vi "Training Top Level.vi"() -> ()   [LabVIEW 2016]
uses:
  Type Definitions/controls_setup.ctl
  Type Definitions/controls_setup_2.ctl
  Type Definitions/control_references.ctl
  <vilib>/Utility/error.llb/DialogType.ctl
panel:
  in  "Water":bool
  in  "Quit":bool=TRUE
  out "Timing Issues":bool
  in  "Config File":path=path "C:/Users/Training/Desktop/TL/lickamundo_amps.ini"
  in  "Base Directory":path=path "C:/Users/Training/Desktop/TL/batch_01_cooling_2"
  in  "Setup 3":bool
  in  "Setup 2":bool
  in  "Setup 1":bool
  in  "Setup 0":bool
  in  "S3":T1={"ChartTemp"=[{"temp in"=32.89921569824219, "temp in"=32.0}, {"temp in"=32.89724349975586, "temp in"=32.0}, {"temp in"=32.890663146972656, "temp in"=32.0}, {"temp in"=32.89329528808594, "temp in"=32.0}, {"temp in"=32.8900032043457, "temp in"=32.0}, {"temp in"=32.88868713378906, "temp in"=32.0}, {"temp in"=32.8900032043457, "temp in"=32.0}, {"temp in"=32.885398864746094, "temp in"=32.0}, {"temp in"=32.88408279418945, "temp in"=32.0}, {"temp in"=32.88079071044922, "temp in"=32.0}, {"temp in"=32.87881851196289, "temp in"=32.0}, {"temp in"=32.87092208862305, "temp in"=32.0}, {"temp in"=32.863685607910156, "temp in"=32.0}, {"temp in"=32.87355422973633, "temp in"=32.0}, {"temp in"=32.87487030029297, "temp in"=32.0}, {"temp in"=32.86763381958008, "temp in"=32.0}, {"temp in"=32.86170959472656, "temp in"=32.0}, {"temp in"=32.858421325683594, "temp in"=32.0}, {"temp in"=32.869606018066406, "temp in"=32.0}, {"temp in"=32.87026596069336, "temp in"=32.0}, {"temp in"=32.865657806396484, "temp in"=32.0}, {"temp in"=32.865657806396484, "temp in"=32.0}, {"temp in"=32.861053466796875, "temp in"=32.0}, {"temp in"=32.863685607910156, "temp in"=32.0}, {"temp in"=32.86170959472656, "temp in"=32.0}, {"temp in"=32.865657806396484, "temp in"=32.0}, {"temp in"=32.862369537353516, "temp in"=32.0}, {"temp in"=32.85578918457031, "temp in"=32.0}, {"temp in"=32.85907745361328, "temp in"=32.0}, {"temp in"=32.8564453125, "temp in"=32.0}, {"temp in"=32.845916748046875, "temp in"=32.0}, {"temp in"=32.85710525512695, "temp in"=32.0}, {"temp in"=32.85249710083008, "temp in"=32.0}, {"temp in"=32.85315704345703, "temp in"=32.0}, {"temp in"=32.85052490234375, "temp in"=32.0}, {"temp in"=32.85447311401367, "temp in"=32.0}, {"temp in"=32.85512924194336, "temp in"=32.0}, {"temp in"=32.86170959472656, "temp in"=32.0}, {"temp in"=32.87487030029297, "temp in"=32.0}, {"temp in"=32.8900032043457, "temp in"=32.0}, {"temp in"=32.906455993652344, "temp in"=32.0}, {"temp in"=32.91303634643555, "temp in"=32.0}, {"temp in"=32.92816925048828, "temp in"=32.0}, {"temp in"=32.93935775756836, "temp in"=32.0}, {"temp in"=32.94659423828125, "temp in"=32.0}, {"temp in"=32.87553024291992, "temp in"=32.0}, {"temp in"=32.891319274902344, "temp in"=32.0}, {"temp in"=32.864341735839844, "temp in"=32.0}, {"temp in"=32.843284606933594, "temp in"=32.0}, {"temp in"=32.844600677490234, "temp in"=32.0}], "ChartLick"=[0.22792984545230865, 0.22776533663272858, 0.22727182507514954, 0.22710731625556946, 0.22644929587841034, 0.2259557843208313, 0.22562678158283234, 0.22529776394367218, 0.22496876120567322, 0.22463975846767426, 0.22463975846767426, 0.2243107408285141, 0.22381722927093506, 0.2234882265329361, 0.22283020615577698, 0.22233669459819794, 0.2218431830406189, 0.2210206538438797, 0.22069165110588074, 0.21986912190914154, 0.21970462799072266, 0.2193756103515625, 0.21888209879398346, 0.21871758997440338, 0.2185530960559845, 0.21805958449840546, 0.2177305668592453, 0.2177305668592453, 0.21756607294082642, 0.21756607294082642, 0.21723705530166626, 0.21674354374408722, 0.21657903492450714, 0.2160855233669281, 0.21592102944850922, 0.21559201180934906, 0.21542751789093018, 0.21542751789093018, 0.21542751789093018, 0.21559201180934906, 0.21625003218650818, 0.21674354374408722, 0.21805958449840546, 0.2193756103515625, 0.22085615992546082, 0.22250120341777802, 0.22365272045135498, 0.2243107408285141, 0.22447524964809418, 0.22447524964809418], "Catch Trials"={"Catch Trials"=0, "Correct Rejections"=0, "False Alarms"=0, "Performance"=100}, "DispStim"={"n"=0, "Hits"=0, "Misses"=0, "Performance"=0}, "Bools"={"Stimulus"=FALSE, "Catch"=FALSE, "Square"=FALSE, "Lick"=FALSE, "Water"=FALSE}, "Time to next stimulus"=0.0, "Recording"=FALSE} {"Time to next stimulus" scale=0.0..1000.0; "DispStim"."Performance" format="%d%%"; "Catch Trials"."Performance" format="%d%%"}
  in  "S2":T1={"ChartTemp"=[{"temp in"=31.964832305908203, "temp in"=32.0}, {"temp in"=31.966148376464844, "temp in"=32.0}, {"temp in"=31.966148376464844, "temp in"=32.0}, {"temp in"=31.970096588134766, "temp in"=32.0}, {"temp in"=31.973386764526367, "temp in"=32.0}, {"temp in"=31.968780517578125, "temp in"=32.0}, {"temp in"=31.968122482299805, "temp in"=32.0}, {"temp in"=31.964174270629883, "temp in"=32.0}, {"temp in"=31.971412658691406, "temp in"=32.0}, {"temp in"=31.969438552856445, "temp in"=32.0}, {"temp in"=31.970096588134766, "temp in"=32.0}, {"temp in"=31.969438552856445, "temp in"=32.0}, {"temp in"=31.970096588134766, "temp in"=32.0}, {"temp in"=31.970096588134766, "temp in"=32.0}, {"temp in"=31.970754623413086, "temp in"=32.0}, {"temp in"=31.972728729248047, "temp in"=32.0}, {"temp in"=31.974044799804688, "temp in"=32.0}, {"temp in"=31.974044799804688, "temp in"=32.0}, {"temp in"=31.972070693969727, "temp in"=32.0}, {"temp in"=31.972728729248047, "temp in"=32.0}, {"temp in"=31.971412658691406, "temp in"=32.0}, {"temp in"=31.970754623413086, "temp in"=32.0}, {"temp in"=31.970754623413086, "temp in"=32.0}, {"temp in"=31.974044799804688, "temp in"=32.0}, {"temp in"=31.972728729248047, "temp in"=32.0}, {"temp in"=31.972728729248047, "temp in"=32.0}, {"temp in"=31.968122482299805, "temp in"=32.0}, {"temp in"=31.968780517578125, "temp in"=32.0}, {"temp in"=31.967464447021484, "temp in"=32.0}, {"temp in"=31.973386764526367, "temp in"=32.0}, {"temp in"=31.970754623413086, "temp in"=32.0}, {"temp in"=31.970096588134766, "temp in"=32.0}, {"temp in"=31.968780517578125, "temp in"=32.0}, {"temp in"=31.968122482299805, "temp in"=32.0}, {"temp in"=31.970754623413086, "temp in"=32.0}, {"temp in"=31.967464447021484, "temp in"=32.0}, {"temp in"=31.969438552856445, "temp in"=32.0}, {"temp in"=31.970096588134766, "temp in"=32.0}, {"temp in"=31.970096588134766, "temp in"=32.0}, {"temp in"=31.968122482299805, "temp in"=32.0}, {"temp in"=31.965490341186523, "temp in"=32.0}, {"temp in"=31.967464447021484, "temp in"=32.0}, {"temp in"=31.966806411743164, "temp in"=32.0}, {"temp in"=31.968780517578125, "temp in"=32.0}, {"temp in"=31.970096588134766, "temp in"=32.0}, {"temp in"=31.965490341186523, "temp in"=32.0}, {"temp in"=31.967464447021484, "temp in"=32.0}, {"temp in"=31.968122482299805, "temp in"=32.0}, {"temp in"=31.968780517578125, "temp in"=32.0}, {"temp in"=31.969438552856445, "temp in"=32.0}], "ChartLick"=[-0.029354939237236977, -0.029354939237236977, -0.029519444331526756, -0.029848452657461166, -0.029848452657461166, -0.030341966077685356, -0.030177460983395576, -0.030506469309329987, -0.030506469309329987, -0.030341966077685356, -0.030670974403619766, -0.030670974403619766, -0.030341966077685356, -0.030506469309329987, -0.030177460983395576, -0.029848452657461166, -0.029848452657461166, -0.029519444331526756, -0.029354939237236977, -0.029354939237236977, -0.029190434142947197, -0.029190434142947197, -0.029354939237236977, -0.029190434142947197, -0.029190434142947197, -0.029519444331526756, -0.029190434142947197, -0.029354939237236977, -0.029354939237236977, -0.029190434142947197, -0.028861425817012787, -0.028861425817012787, -0.029025930911302567, -0.029190434142947197, -0.029025930911302567, -0.029354939237236977, -0.029354939237236977, -0.029519444331526756, -0.029683947563171387, -0.029519444331526756, -0.029354939237236977, -0.029354939237236977, -0.029190434142947197, -0.029190434142947197, -0.029190434142947197, -0.028861425817012787, -0.029354939237236977, -0.029354939237236977, -0.029519444331526756, -0.029683947563171387], "Catch Trials"={"Catch Trials"=0, "Correct Rejections"=0, "False Alarms"=0, "Performance"=100}, "DispStim"={"n"=0, "Hits"=0, "Misses"=0, "Performance"=0}, "Bools"={"Stimulus"=FALSE, "Catch"=FALSE, "Square"=FALSE, "Lick"=FALSE, "Water"=FALSE}, "Time to next stimulus"=0.0, "Recording"=FALSE} {"Time to next stimulus" scale=0.0..1000.0; "DispStim"."Performance" format="%d%%"; "Catch Trials"."Performance" format="%d%%"}
  in  "S1":T1={"ChartTemp"=[{"temp in"=31.926668167114258, "temp in"=32.0}, {"temp in"=31.93785285949707, "temp in"=32.0}, {"temp in"=31.93456268310547, "temp in"=32.0}, {"temp in"=31.926668167114258, "temp in"=32.0}, {"temp in"=31.92930030822754, "temp in"=32.0}, {"temp in"=31.926010131835938, "temp in"=32.0}, {"temp in"=31.93587875366211, "temp in"=32.0}, {"temp in"=31.927326202392578, "temp in"=32.0}, {"temp in"=31.93719482421875, "temp in"=32.0}, {"temp in"=31.92995834350586, "temp in"=32.0}, {"temp in"=31.947065353393555, "temp in"=32.0}, {"temp in"=31.92995834350586, "temp in"=32.0}, {"temp in"=31.92864227294922, "temp in"=32.0}, {"temp in"=31.93653678894043, "temp in"=32.0}, {"temp in"=31.93785285949707, "temp in"=32.0}, {"temp in"=31.93390655517578, "temp in"=32.0}, {"temp in"=31.93456268310547, "temp in"=32.0}, {"temp in"=31.93851089477539, "temp in"=32.0}, {"temp in"=31.93916893005371, "temp in"=32.0}, {"temp in"=31.93522071838379, "temp in"=32.0}, {"temp in"=31.93193244934082, "temp in"=32.0}, {"temp in"=31.93456268310547, "temp in"=32.0}, {"temp in"=31.93785285949707, "temp in"=32.0}, {"temp in"=31.93916893005371, "temp in"=32.0}, {"temp in"=31.94048500061035, "temp in"=32.0}, {"temp in"=31.944433212280273, "temp in"=32.0}, {"temp in"=31.945749282836914, "temp in"=32.0}, {"temp in"=31.93390655517578, "temp in"=32.0}, {"temp in"=31.93324851989746, "temp in"=32.0}, {"temp in"=31.941143035888672, "temp in"=32.0}, {"temp in"=31.941143035888672, "temp in"=32.0}, {"temp in"=31.945091247558594, "temp in"=32.0}, {"temp in"=31.93851089477539, "temp in"=32.0}, {"temp in"=31.93061637878418, "temp in"=32.0}, {"temp in"=31.93587875366211, "temp in"=32.0}, {"temp in"=31.925352096557617, "temp in"=32.0}, {"temp in"=31.941143035888672, "temp in"=32.0}, {"temp in"=31.947723388671875, "temp in"=32.0}, {"temp in"=31.946407318115234, "temp in"=32.0}, {"temp in"=31.93916893005371, "temp in"=32.0}, {"temp in"=31.942459106445312, "temp in"=32.0}, {"temp in"=31.93916893005371, "temp in"=32.0}, {"temp in"=31.93916893005371, "temp in"=32.0}, {"temp in"=31.93785285949707, "temp in"=32.0}, {"temp in"=31.93259048461914, "temp in"=32.0}, {"temp in"=31.947065353393555, "temp in"=32.0}, {"temp in"=31.94048500061035, "temp in"=32.0}, {"temp in"=31.94048500061035, "temp in"=32.0}, {"temp in"=31.93522071838379, "temp in"=32.0}, {"temp in"=31.93851089477539, "temp in"=32.0}], "ChartLick"=[-0.015372068621218204, 0.008645567111670971, 0.010455114766955376, 0.01226466242223978, 0.01308718416839838, 0.32400035858154297, 0.4118456542491913, 0.3945727050304413, 0.2456963062286377, 0.11310582607984543, 0.023286454379558563, -0.004679285921156406, -0.002376224845647812, -0.0031987465918064117, -0.0033632509876042604, -0.30802538990974426, -0.4100181758403778, -0.41363725066185, -0.26953136920928955, -0.12542548775672913, -0.01553657278418541, 0.008810071274638176, 0.01111313235014677, 0.012100158259272575, 0.012100158259272575, 0.32498738169670105, 0.4116811454296112, 0.3906245827674866, 0.24306423962116241, 0.11491537094116211, 0.021312402561306953, -0.004514781292527914, -0.0027052334044128656, -0.002540729008615017, -0.0033632509876042604, -0.3095059394836426, -0.4108406901359558, -0.4123212397098541, -0.2677218019962311, -0.12493197619915009, -0.015207564458251, 0.008645567111670971, 0.011277636513113976, 0.012100158259272575, 0.012429166585206985, 0.3287709653377533, 0.40970709919929504, 0.3934211730957031, 0.24372224509716034, 0.11195429414510727], "Catch Trials"={"Catch Trials"=135, "Correct Rejections"=0, "False Alarms"=135, "Performance"=0}, "DispStim"={"n"=136, "Hits"=136, "Misses"=0, "Performance"=100}, "Bools"={"Stimulus"=FALSE, "Catch"=FALSE, "Square"=FALSE, "Lick"=FALSE, "Water"=FALSE}, "Time to next stimulus"=20000.0, "Recording"=FALSE} caption="Setup 1" {"Time to next stimulus" scale=0.0..20000.0; "DispStim"."Performance" format="%d%%"; "Catch Trials"."Performance" format="%d%%"}
  in  "S0":T1={"ChartTemp"=[{"temp in"=31.942459106445312, "temp in"=32.0}, {"temp in"=31.951013565063477, "temp in"=32.0}, {"temp in"=31.949697494506836, "temp in"=32.0}, {"temp in"=31.949039459228516, "temp in"=32.0}, {"temp in"=31.951013565063477, "temp in"=32.0}, {"temp in"=31.950355529785156, "temp in"=32.0}, {"temp in"=31.95890998840332, "temp in"=32.0}, {"temp in"=31.944433212280273, "temp in"=32.0}, {"temp in"=31.952987670898438, "temp in"=32.0}, {"temp in"=31.945749282836914, "temp in"=32.0}, {"temp in"=31.92995834350586, "temp in"=32.0}, {"temp in"=31.954303741455078, "temp in"=32.0}, {"temp in"=31.943117141723633, "temp in"=32.0}, {"temp in"=31.95956802368164, "temp in"=32.0}, {"temp in"=31.962858200073242, "temp in"=32.0}, {"temp in"=31.9615421295166, "temp in"=32.0}, {"temp in"=31.9615421295166, "temp in"=32.0}, {"temp in"=31.9615421295166, "temp in"=32.0}, {"temp in"=31.962200164794922, "temp in"=32.0}, {"temp in"=31.966148376464844, "temp in"=32.0}, {"temp in"=31.96088409423828, "temp in"=32.0}, {"temp in"=31.95759391784668, "temp in"=32.0}, {"temp in"=31.954303741455078, "temp in"=32.0}, {"temp in"=31.962858200073242, "temp in"=32.0}, {"temp in"=31.962200164794922, "temp in"=32.0}, {"temp in"=31.952329635620117, "temp in"=32.0}, {"temp in"=31.94048500061035, "temp in"=32.0}, {"temp in"=31.95759391784668, "temp in"=32.0}, {"temp in"=31.952987670898438, "temp in"=32.0}, {"temp in"=31.966806411743164, "temp in"=32.0}, {"temp in"=31.958251953125, "temp in"=32.0}, {"temp in"=31.95890998840332, "temp in"=32.0}, {"temp in"=31.962858200073242, "temp in"=32.0}, {"temp in"=31.95956802368164, "temp in"=32.0}, {"temp in"=31.9549617767334, "temp in"=32.0}, {"temp in"=31.9549617767334, "temp in"=32.0}, {"temp in"=31.964174270629883, "temp in"=32.0}, {"temp in"=31.95759391784668, "temp in"=32.0}, {"temp in"=31.962858200073242, "temp in"=32.0}, {"temp in"=31.96088409423828, "temp in"=32.0}, {"temp in"=31.95759391784668, "temp in"=32.0}, {"temp in"=31.95627784729004, "temp in"=32.0}, {"temp in"=31.966806411743164, "temp in"=32.0}, {"temp in"=31.95693588256836, "temp in"=32.0}, {"temp in"=31.95890998840332, "temp in"=32.0}, {"temp in"=31.966148376464844, "temp in"=32.0}, {"temp in"=31.96088409423828, "temp in"=32.0}, {"temp in"=31.95627784729004, "temp in"=32.0}, {"temp in"=31.972070693969727, "temp in"=32.0}, {"temp in"=31.958251953125, "temp in"=32.0}], "ChartLick"=[-0.019978191703557968, 0.008974575437605381, 0.010948628187179565, 0.011771149933338165, 0.013251688331365585, 0.32021674513816833, 0.41299718618392944, 0.39555972814559937, 0.2440512627363205, 0.11524438112974167, 0.021147897467017174, -0.0050082942470908165, -0.0027052334044128656, -0.003034242196008563, -0.0033632509876042604, -0.3034192621707916, -0.4126502275466919, -0.4157758355140686, -0.2718344032764435, -0.1272350400686264, -0.01586558111011982, 0.008481062948703766, 0.010948628187179565, 0.011771149933338165, 0.01275817584246397, 0.3190652132034302, 0.4125036597251892, 0.39309215545654297, 0.24207721650600433, 0.11606690287590027, 0.023286454379558563, -0.004514781292527914, -0.002376224845647812, -0.0028697378002107143, -0.003692259546369314, -0.3075318932533264, -0.4108406901359558, -0.41314375400543213, -0.266734778881073, -0.12855108082294464, -0.01553657278418541, 0.008974575437605381, 0.01111313235014677, 0.011771149933338165, 0.012429166585206985, 0.32416486740112305, 0.4106941223144531, 0.3934211730957031, 0.2448737770318985, 0.11343482881784439], "Catch Trials"={"Catch Trials"=115, "Correct Rejections"=0, "False Alarms"=115, "Performance"=0}, "DispStim"={"n"=116, "Hits"=116, "Misses"=0, "Performance"=100}, "Bools"={"Stimulus"=FALSE, "Catch"=FALSE, "Square"=FALSE, "Lick"=FALSE, "Water"=FALSE}, "Time to next stimulus"=20000.0, "Recording"=FALSE} {"Time to next stimulus" scale=0.0..20000.0; "DispStim"."Performance" format="%d%%"; "Catch Trials"."Performance" format="%d%%"}
  in  "Setup 3 Controls":T2={"Animal"=4, "Session"=1, "Free Reward"=FALSE, "Start"=FALSE, "Pause"=FALSE, "Stop"=FALSE} {"Session" min=1 step=1 format="%03.0f"; "Animal" min=1 step=1 format="%03.0f"}
  in  "Setup 2 Controls":T2={"Animal"=3, "Session"=2, "Free Reward"=FALSE, "Start"=FALSE, "Pause"=FALSE, "Stop"=FALSE} {"Session" min=1 step=1 format="%03.0f"; "Animal" min=1 step=1 format="%03.0f"}
  in  "Setup 1 Controls":T2={"Animal"=2, "Session"=6, "Free Reward"=FALSE, "Start"=FALSE, "Pause"=FALSE, "Stop"=FALSE} {"Session" min=1 step=1 format="%03.0f"; "Animal" min=1 step=1 format="%03.0f"}
  in  "Setup 0 Controls":T2={"Animal"=3, "Session"=3, "Free Reward"=FALSE, "Start"=FALSE, "Pause"=FALSE, "Stop"=FALSE} {"Session" min=1 step=1 format="%03.0f"; "Animal" min=1 step=1 format="%03.0f"}
  # "Animal Training"
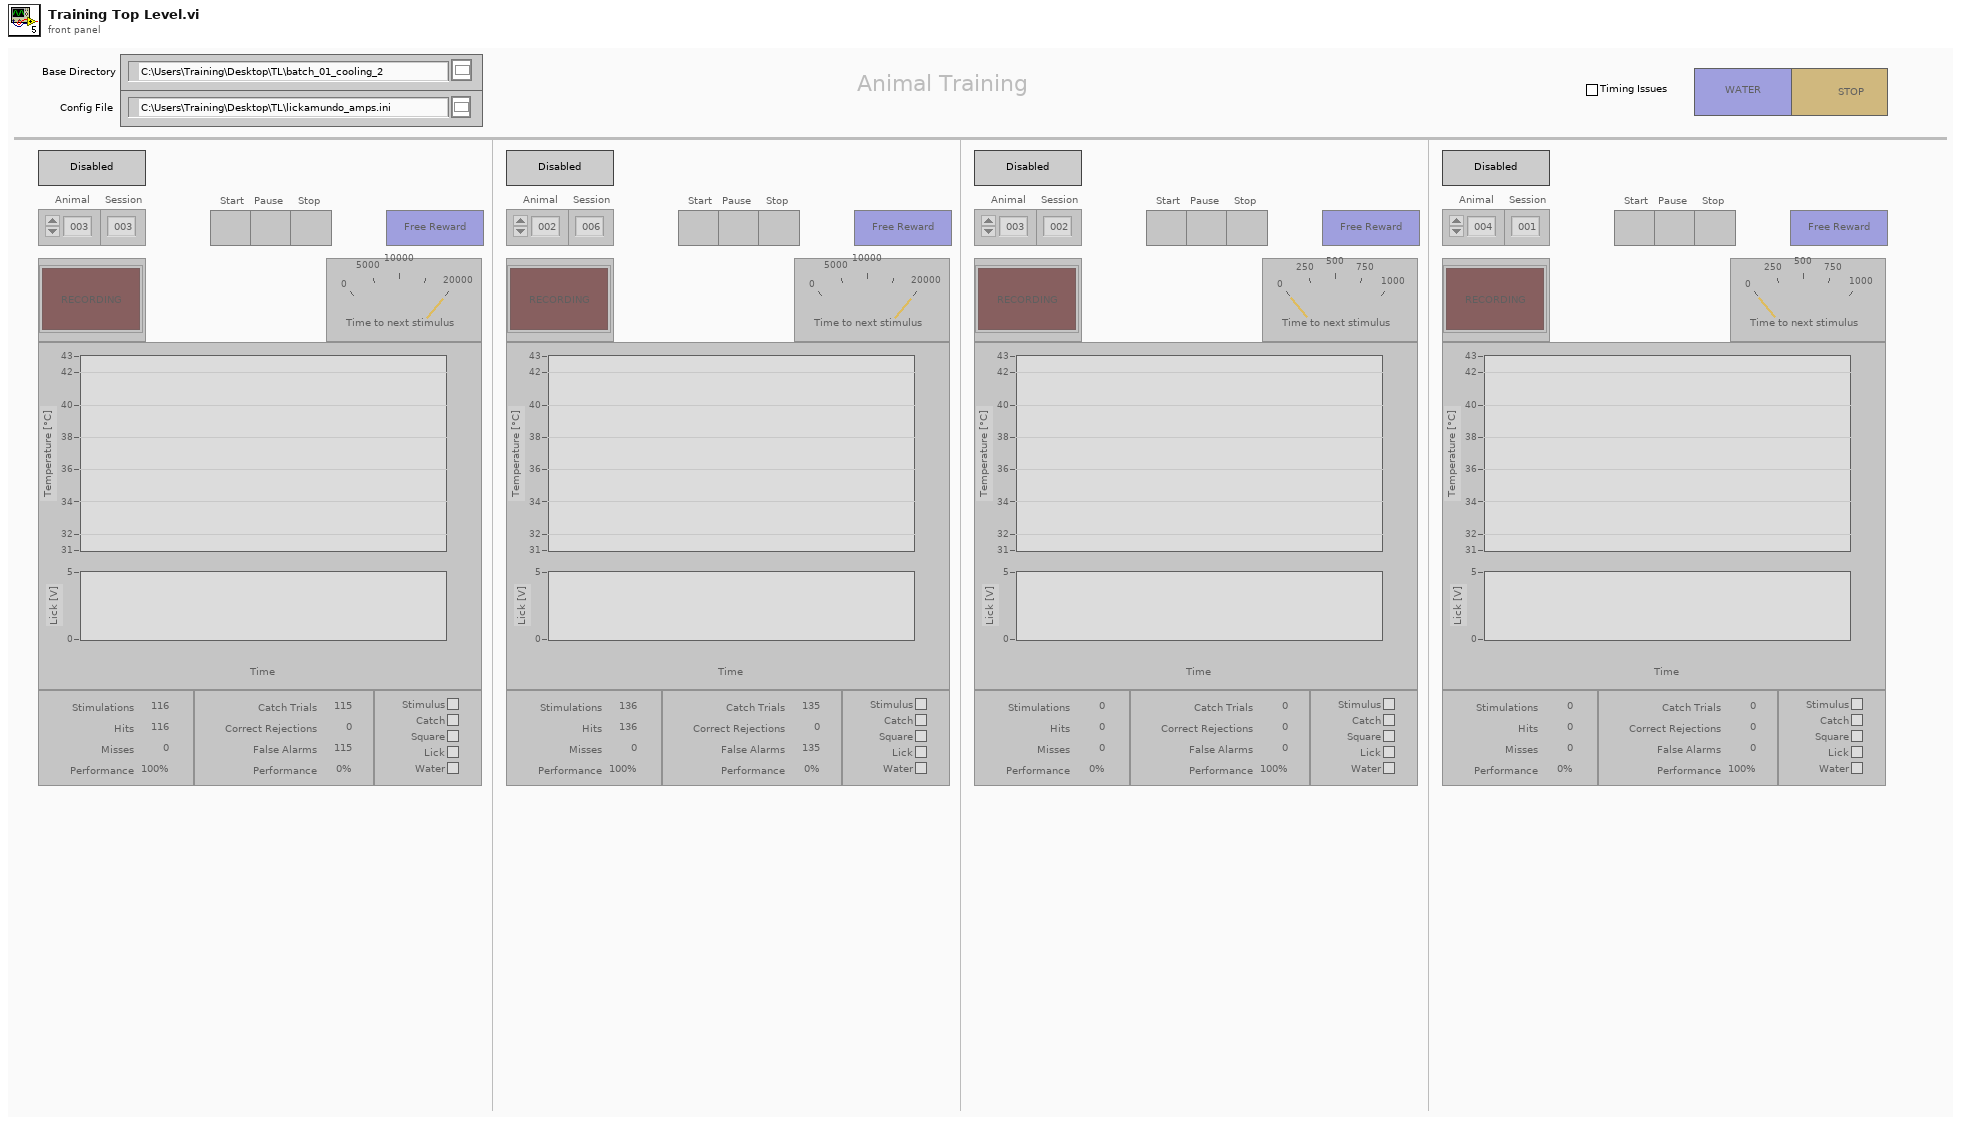
[diagram p1: front panel]
types:
  T1 = typedef "controls_setup.ctl" = cluster{"ChartTemp":cluster{"temp in":dbl, "temp in":dbl}[], "ChartLick":dbl[], "Catch Trials":cluster{"Catch Trials":u16, "Correct Rejections":u16, "False Alarms":u16, "Performance":u16}, "DispStim":cluster{"n":u16, "Hits":u16, "Misses":u16, "Performance":u16}, "Bools":cluster{"Stimulus":bool, "Catch":bool, "Square":bool, "Lick":bool, "Water":bool}, "Time to next stimulus":dbl, "Recording":bool}
  T2 = typedef "controls_setup_2.ctl" = cluster{"Animal":u16, "Session":u16, "Free Reward":bool, "Start":bool, "Pause":bool, "Stop":bool}
  T3 = typedef "DialogType.ctl" = u16
  T4 = typedef "control_references.ctl" = cluster{"Base Directory":refnum<vi>, "Config File":refnum<vi>, "Timing Issues":refnum<vi>, "Quit":refnum<vi>, "Animal ID":refnum<vi>[], "Session ID":refnum<vi>[], "Active":refnum<vi>[], "Temperature Charts":refnum<vi>[], "Lick Charts":refnum<vi>[], "Bool Displays":refnum<vi>[], "Stimulus Timing":refnum<vi>[], "Stimulus Stats":refnum<vi>[], "Catch Stats":refnum<vi>[], "Recording Status":refnum<vi>[]}
  T5 = typedef "reference_cluster.ctl" = cluster{"Vars":cluster{"General":refnum<notifier>, "Runtime":refnum<notifier>}, "Data":cluster{"Display":refnum<queue>, "Write":refnum<queue>}, "LoopCtrl":cluster{"Display":refnum<notifier>, "DAQ":refnum<notifier>, "Write":refnum<notifier>[]}, "Controls":T4, "Error Event":refnum<user-event>}
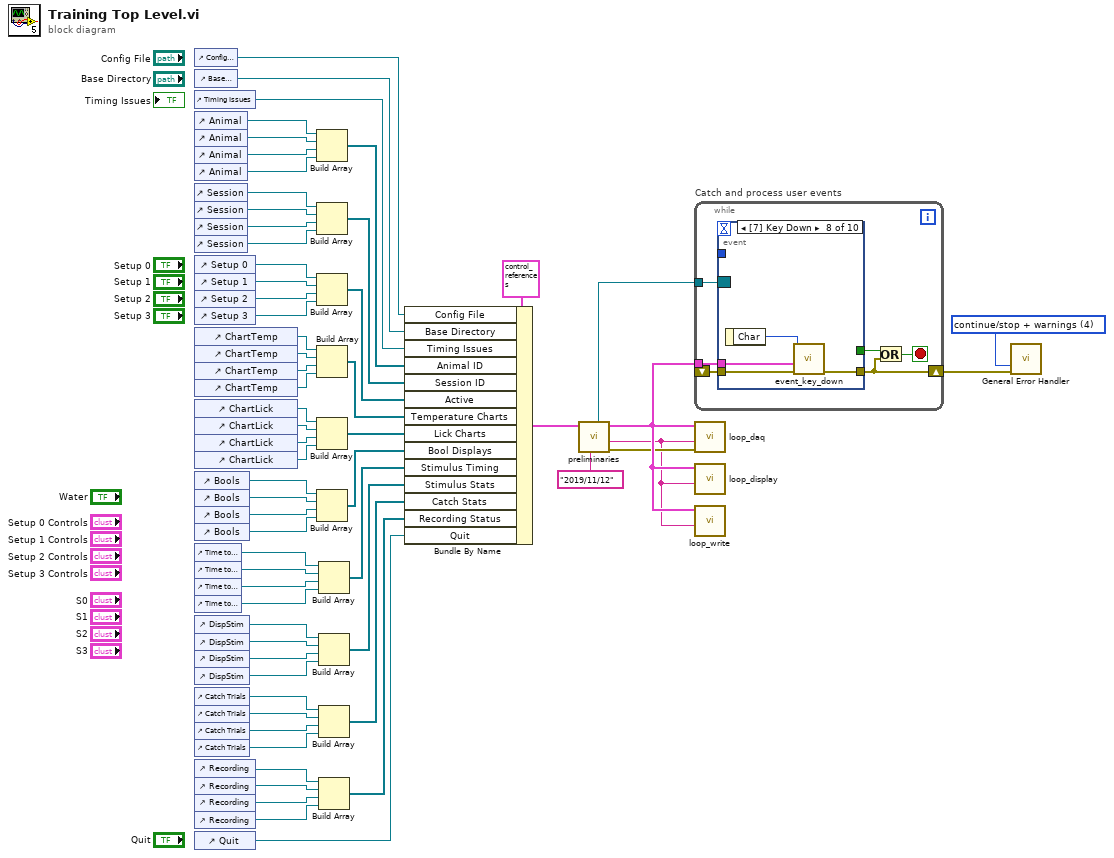
[diagram p0: block diagram]
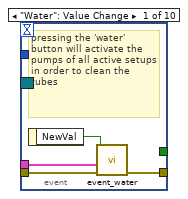
[diagram p2: hidden frame]
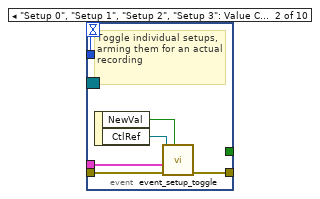
[diagram p3: hidden frame]
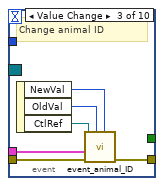
[diagram p4: hidden frame]
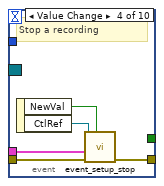
[diagram p5: hidden frame]
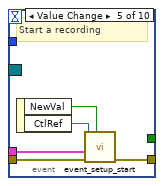
[diagram p6: hidden frame]
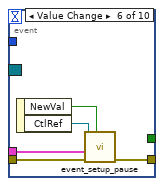
[diagram p7: hidden frame]
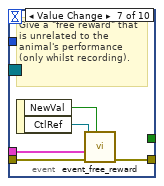
[diagram p8: hidden frame]
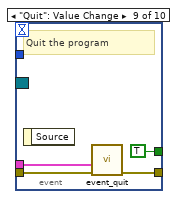
[diagram p9: hidden frame]
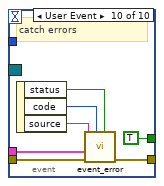
[diagram p10: hidden frame]
diagram:
  w10 = T3 4 items=["no dialog", "OK message", "continue or stop message", "OK message + warnings", "continue/stop + warnings"] ("type of dialog (OK msg:1)")
  n1 = control-ref of="Config File"() -> (w13:refnum<vi>)
  n2 = control-ref of="Base Directory"() -> (w38:refnum<vi>)
  n3 = control-ref of="Timing Issues"() -> (w39:refnum<vi>)
  n4 = control-ref of="Animal"() -> (w37:refnum<vi>)
  n5 = control-ref of="Animal"() -> (w36:refnum<vi>)
  n6 = control-ref of="Animal"() -> (w35:refnum<vi>)
  n7 = control-ref of="Animal"() -> (w34:refnum<vi>)
  n8 = control-ref of="Session"() -> (w33:refnum<vi>)
  n9 = control-ref of="Session"() -> (w32:refnum<vi>)
  n10 = control-ref of="Session"() -> (w31:refnum<vi>)
  n11 = control-ref of="Session"() -> (w30:refnum<vi>)
  n12 = control-ref of="Setup 0"() -> (w29:refnum<vi>)
  n13 = control-ref of="Setup 1"() -> (w28:refnum<vi>)
  n14 = control-ref of="Setup 2"() -> (w27:refnum<vi>)
  n15 = control-ref of="Setup 3"() -> (w26:refnum<vi>)
  n16 = control-ref of="ChartTemp"() -> (w62:refnum<vi>)
  n17 = control-ref of="ChartTemp"() -> (w61:refnum<vi>)
  n18 = control-ref of="ChartTemp"() -> (w60:refnum<vi>)
  n19 = control-ref of="ChartTemp"() -> (w59:refnum<vi>)
  n20 = control-ref of="ChartLick"() -> (w58:refnum<vi>)
  n21 = control-ref of="ChartLick"() -> (w55:refnum<vi>)
  n22 = control-ref of="ChartLick"() -> (w56:refnum<vi>)
  n23 = control-ref of="ChartLick"() -> (w57:refnum<vi>)
  n24 = control-ref of="Bools"() -> (w54:refnum<vi>)
  n25 = control-ref of="Bools"() -> (w51:refnum<vi>)
  n26 = control-ref of="Bools"() -> (w52:refnum<vi>)
  n27 = control-ref of="Bools"() -> (w53:refnum<vi>)
  n28 = control-ref of="Time to next stimulus"() -> (w50:refnum<vi>)
  n29 = control-ref of="Time to next stimulus"() -> (w47:refnum<vi>)
  n30 = control-ref of="Time to next stimulus"() -> (w48:refnum<vi>)
  n31 = control-ref of="Time to next stimulus"() -> (w49:refnum<vi>)
  n32 = control-ref of="DispStim"() -> (w25:refnum<vi>)
  n33 = control-ref of="DispStim"() -> (w23:refnum<vi>)
  n34 = control-ref of="DispStim"() -> (w22:refnum<vi>)
  n35 = control-ref of="DispStim"() -> (w24:refnum<vi>)
  n36 = control-ref of="Catch Trials"() -> (w18:refnum<vi>)
  n37 = control-ref of="Catch Trials"() -> (w20:refnum<vi>)
  n38 = control-ref of="Catch Trials"() -> (w21:refnum<vi>)
  n39 = control-ref of="Catch Trials"() -> (w19:refnum<vi>)
  n40 = control-ref of="Recording"() -> (w9:refnum<vi>)
  n41 = control-ref of="Recording"() -> (w8:refnum<vi>)
  n42 = control-ref of="Recording"() -> (w7:refnum<vi>)
  n43 = control-ref of="Recording"() -> (w6:refnum<vi>)
  n44 = control-ref of="Quit"() -> (w12:refnum<vi>)
  n45 = Build Array(w37, w36, w35, w34) -> (w40:refnum<vi>[])
  n46 = Build Array(w33, w32, w31, w30) -> (w41:refnum<vi>[])
  n47 = Build Array(w29, w28, w27, w26) -> (w44:refnum<vi>[])
  n48 = Build Array(w62, w61, w60, w59) -> (w46:refnum<vi>[])
  n49 = Build Array(w58, w55, w56, w57) -> (w45:refnum<vi>[])
  n50 = Build Array(w54, w51, w52, w53) -> (w14:refnum<vi>[])
  n51 = Build Array(w50, w47, w48, w49) -> (w43:refnum<vi>[])
  n52 = Build Array(w25, w23, w22, w24) -> (w17:refnum<vi>[])
  n53 = Build Array(w18, w20, w21, w19) -> (w16:refnum<vi>[])
  n54 = Build Array(w9, w8, w7, w6) -> (w15:refnum<vi>[])
  n55 = Bundle By Name(cluster=T4 {"Base Directory"=refnum, "Config File"=refnum, "Timing Issues"=refnum, "Quit"=refnum, "Animal ID"=[], "Session ID"=[], "Active"=[], "Temperature Charts"=[], "Lick Charts"=[], "Bool Displays"=[], "Stimulus Timing"=[], "Stimulus Stats"=[], "Catch Stats"=[], "Recording Status"=[]} ("Cluster"), "Config File"=w13, "Base Directory"=w38, "Timing Issues"=w39, "Animal ID"=w40, "Session ID"=w41, "Active"=w44, "Temperature Charts"=w46, "Lick Charts"=w45, "Bool Displays"=w14, "Stimulus Timing"=w43, "Stimulus Stats"=w17, "Catch Stats"=w16, "Recording Status"=w15, "Quit"=w12) -> (w1:T4)
  n56 = call "preliminaries.vi"("Version"="2019/11/12" ("Last modified"), "control cluster"=w1) -> ("error out"=w5:errorcluster, "timing source out"=w4:string, "reference cluster out"=w63:T5, "error event refnum"=w2:refnum<event-registration>)  [unwired: 4 in]
  n57 = while "Catch and process user events" {
    shift-right: [w65] -> w11
    shift-left: _ -> [w69]
    tunnel: w63 -> [w68]
    tunnel: w2 -> [w64]
    stop <- w67 stop-if-true
    n58 = event shown="[7] Key Down" {
      selector: w64 -> [_ _ _ _ _ _ _ _ _ _]
      dyn-events: _ -> [_ _ _ _ _ _ _ _ _ _]
      timeout: _ -> [_ w74 _ _ _ _ _ _ _ _]
      tunnel: [_ _ _ _ _ _ _ _ TRUE TRUE] -> w66
      tunnel: w69 -> [w72 w76 w85 w88 w93 w99 w105 w109 w112 w119]
      tunnel: [w73 w79 w84 w90 w95 w98 w104 w108 w111 w120] -> w65
      tunnel: w68 -> [w71 w78 w80 w89 w94 w100 w103 w106 w110 w118]
      tunnel: [_ w74 _ _ _ _ _ _ _ _] -> _
      event "Water": Value Change {
        # "pressing the 'water' button will activate the pumps of all active setups in order to clean the tubes"
        n59 = event-data() -> ("NewVal"=w70:bool)  [unwired: 1 in]
        n60 = call "event_water.vi"("error in"=w72, "reference cluster in"=w71, "water on?"=w70) -> ("error out"=w73:errorcluster)  [unwired: 8 in]
      }
      event "Setup 0", "Setup 1", "Setup 2", "Setup 3": Value Change {
        # "Toggle individual setups, arming them for an actual recording"
        n61 = event-data() -> ("NewVal"=w75:bool, "CtlRef"=w77:refnum<vi>)  [unwired: 1 in]
        n62 = call "event_setup_toggle.vi"("NewVal"=w75, "error in"=w76, "reference cluster in"=w78, "Boolean in"=w77) -> ("error out"=w79:errorcluster)  [unwired: 7 in]
      }
      event Value Change {
        # "Change animal ID"
        n63 = event-data() -> ("NewVal"=w81:u16, "OldVal"=w82:u16, "CtlRef"=w83:refnum<vi>)  [unwired: 1 in]
        n64 = call "event_animal_ID.vi"("NewVal"=w81, "OldVal"=w82, "error in"=w85, "reference cluster in"=w80, "Digital in"=w83) -> ("error out"=w84:errorcluster)  [unwired: 6 in]
      }
      event Value Change {
        # "Stop a recording"
        n65 = event-data() -> ("NewVal"=w86:bool, "CtlRef"=w87:refnum<vi>)  [unwired: 1 in]
        n66 = call "event_setup_stop.vi"("NewVal"=w86, "error in (no error)"=w88, "reference cluster in"=w89, "Boolean in"=w87) -> ("error out"=w90:errorcluster)  [unwired: 7 in]
      }
      event Value Change {
        # "Start a recording"
        n67 = event-data() -> ("NewVal"=w91:bool, "CtlRef"=w92:refnum<vi>)  [unwired: 1 in]
        n68 = call "event_setup_start.vi"("NewVal"=w91, "error in"=w93, "reference cluster in"=w94, "Boolean in"=w92) -> ("error out"=w95:errorcluster)  [unwired: 7 in]
      }
      event Value Change {
        n69 = event-data() -> ("NewVal"=w96:bool, "CtlRef"=w97:refnum<vi>)  [unwired: 1 in]
        n70 = call "event_setup_pause.vi"("NewVal"=w96, "error in"=w99, "reference cluster in"=w100, "Boolean in"=w97) -> ("error out"=w98:errorcluster)  [unwired: 7 in]
      }
      event Value Change {
        # "Give a \"free reward\" that is unrelated to the animal's performance (only whilst recording)."
        n71 = event-data() -> ("NewVal"=w101:bool, "CtlRef"=w102:refnum<vi>)  [unwired: 1 in]
        n72 = call "event_free_reward.vi"("New Value"=w101, "error in"=w105, "reference cluster in"=w103, "CtrLRef"=w102) -> ("error out"=w104:errorcluster)  [unwired: 7 in]
      }
      event Key Down {
        n73 = event-data() -> ("Char"=w107:i16)  [unwired: 1 in]
        n74 = call "event_key_down.vi"("error in"=w109, "reference cluster in"=w106, "Char"=w107) -> ("error out"=w108:errorcluster)  [unwired: 8 in]
      }
      event "Quit": Value Change {
        # "Quit the program"
        n75 = event-data() -> ()  [unwired: 1 in, 1 out]
        n76 = call "event_quit.vi"("error in"=w112, "reference cluster in"=w110) -> ("error out"=w111:errorcluster)  [unwired: 9 in]
      }
      event User Event {
        # "catch errors"
        n77 = event-data() -> ("status"=w117:bool, "code"=w116:i32, "source"=w115:string)  [unwired: 1 in]
        n78 = call "event_error.vi"("status"=w117, "code"=w116, "error in"=w119, "reference cluster"=w118, "source"=w115) -> ("error out"=w120:errorcluster)  [unwired: 6 in]
      }
    }
    n79 = Or(x=w66, y=w65) -> (x .or. y?=w67:bool)
  }
  n80 = call "loop_daq.vi"("error in"=w5, "timing source"=w4, "reference cluster"=w63) -> ()  [unwired: 9 in]
  n81 = call "loop_display.vi"("timing source"=w4, "reference cluster"=w63) -> ()  [unwired: 10 in]
  n82 = call "loop_write.vi"("timing source"=w4, "reference cluster"=w63) -> ()  [unwired: 10 in]
  n83 = call <vilib>:"General Error Handler.vi"("type of dialog (OK msg:1)"=w10, "error in (no error)"=w11) -> ()  [unwired: 9 in, 5 out]
